vi "Get Screenshots.vi"(8 "error in (no error)":errorcluster, 10 "Screenshot Type":T3, 11 "VI Screenshots In":T1) -> (0 "error out":errorcluster, 2 "Screenshot Paths":path[](array[path]))   [LabVIEW 2015, in "VIDiff_Screenshots.lvlib"]
uses:
  VIDiff_Screenshots.lvlib
  Screenshot Type.ctl
  VI Screenshots.ctl
  Screenshot Info.ctl
  Utilities/FilePaths.ctl
  utilities/VIDiff_Utilities.lvlib
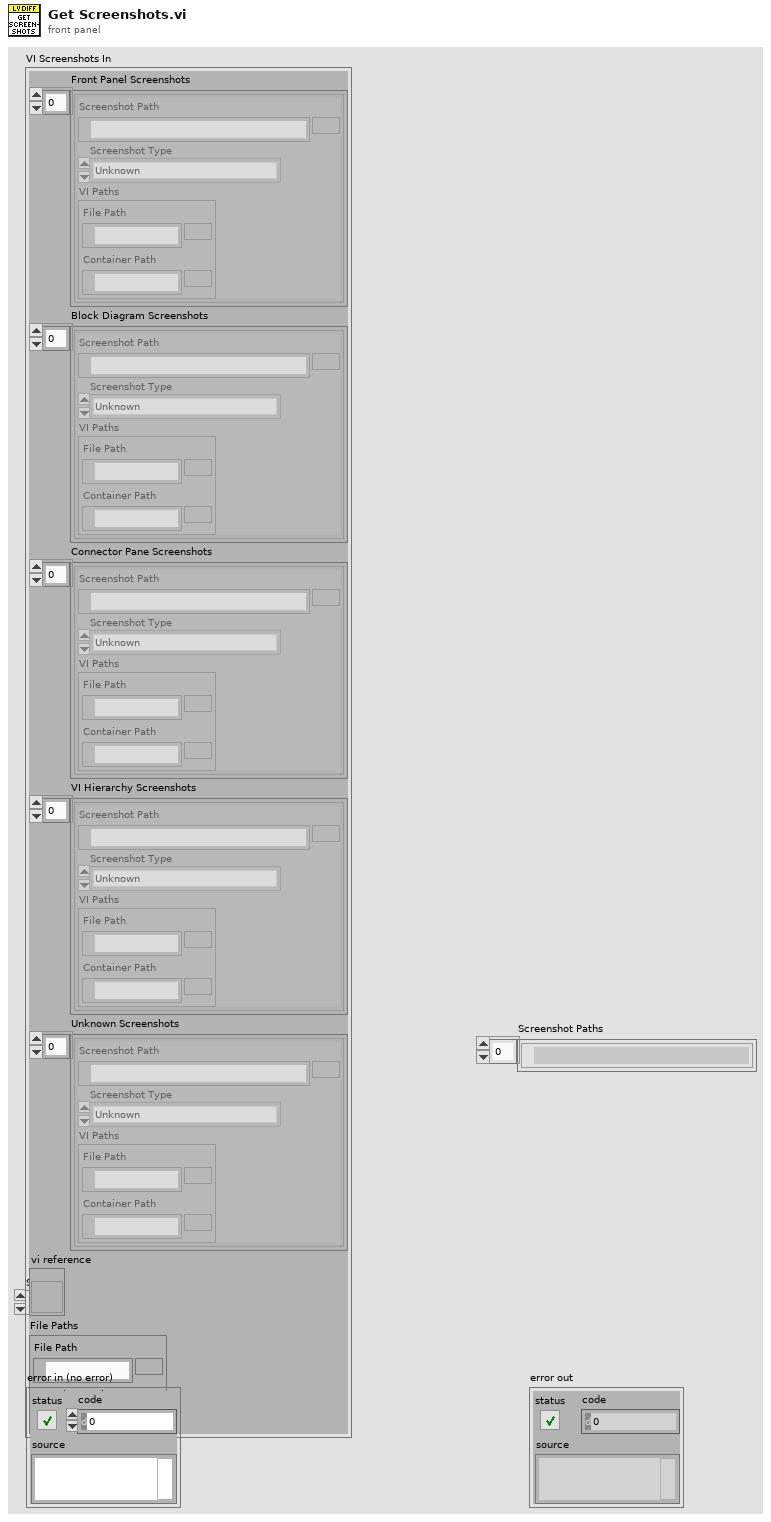
[diagram p1: front panel]
types:
  T1 = typedef "VIDiff_Screenshots.lvlib/VI Screenshots.ctl" = cluster{"Front Panel Screenshots":T2[], "Block Diagram Screenshots":T2[], "Connector Pane Screenshots":T2[], "VI Hierarchy Screenshots":T2[], "Unknown Screenshots":T2[], "vi reference":refnum<vi>, "File Paths":cluster{"File Path":path, "Container Path":path}}
  T2 = typedef "VIDiff_Screenshots.lvlib/Screenshot Info.ctl" = cluster{"Screenshot Path":path, "Screenshot Type":T3, "VI Paths":T4}
  T3 = typedef "VIDiff_Screenshots.lvlib/Screenshot Type.ctl" = enum16{"Unknown", "Front Panel", "Connector Pane", "Block Diagram", "VI Hierarchy"}
  T4 = typedef "VIDiff_Utilities.lvlib/FilePaths.ctl" = cluster{"File Path":path, "Container Path":path}
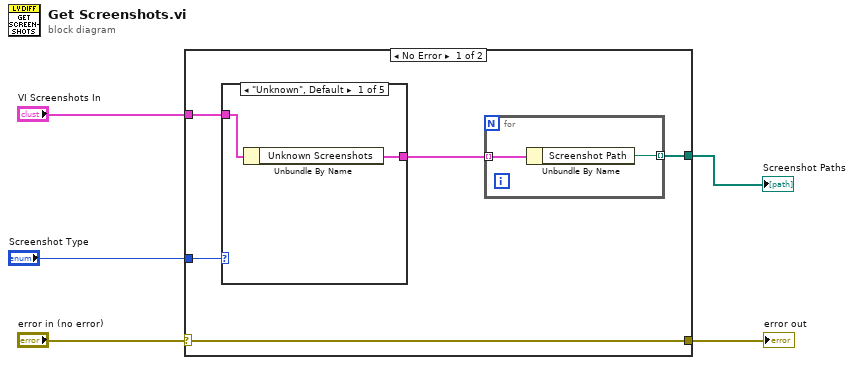
[diagram p0: block diagram]
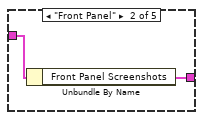
[diagram p2: hidden frame]
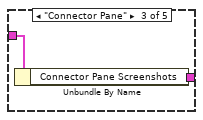
[diagram p3: hidden frame]
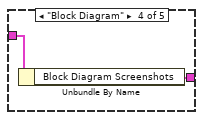
[diagram p4: hidden frame]
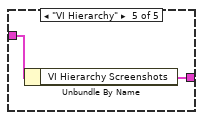
[diagram p5: hidden frame]
diagram:
  n1 = case shown="No Error" "error in (no error)" {
    selector: "error in (no error)" -> [w10 w23]
    tunnel: [w10 w23] -> w4
    tunnel: "VI Screenshots In" -> [w8 _]
    tunnel: "Screenshot Type" -> [w9 _]
    tunnel: [w6 _] -> w1
    frame No Error {
      n2 = case shown="\"Unknown\", Default" w9 {
        tunnel: w8 -> [w12 w14 w16 w18 w20]
        tunnel: [w11 w13 w15 w17 w19] -> w7
        frame "Unknown", Default {
          n3 = Unbundle By Name(w12) -> ("Unknown Screenshots"=w11:T2[])
        }
        frame "Front Panel" {
          n4 = Unbundle By Name(w14) -> ("Front Panel Screenshots"=w13:T2[])
        }
        frame "Connector Pane" {
          n5 = Unbundle By Name(w16) -> ("Connector Pane Screenshots"=w15:T2[])
        }
        frame "Block Diagram" {
          n6 = Unbundle By Name(w18) -> ("Block Diagram Screenshots"=w17:T2[])
        }
        frame "VI Hierarchy" {
          n7 = Unbundle By Name(w20) -> ("VI Hierarchy Screenshots"=w19:T2[])
        }
      }
      n8 = for {
        tunnel: w7 -> [w22] mode=indexing
        tunnel: [w21] -> w6 mode=indexing
        n9 = Unbundle By Name(w22) -> ("Screenshot Path"=w21:path)
      }
    }
    frame Error {
    }
  }
  "error out" <- w4
  "Screenshot Paths" <- w1
